vi "Load Normalised ROI setup values file.vi"(11 "Experiment data folder path":path) -> (1 "Normalised ROI file data size":i32[](array[numeric]), 2 "Normalised ROI file data (header removed)":dbl[][](array[numeric]), 3 "Norm ROI columns header":string[](array[string]), 5 "Version index (-1 = latest version)":i32)   [LabVIEW 2017]
uses:
  Typedefs/Enum-Which file or folder.ctl
  <userlib>/My Palettes.lib/Files & paths/Spreadsheet/Read From Spreadsheet File (string)-Mod.vi
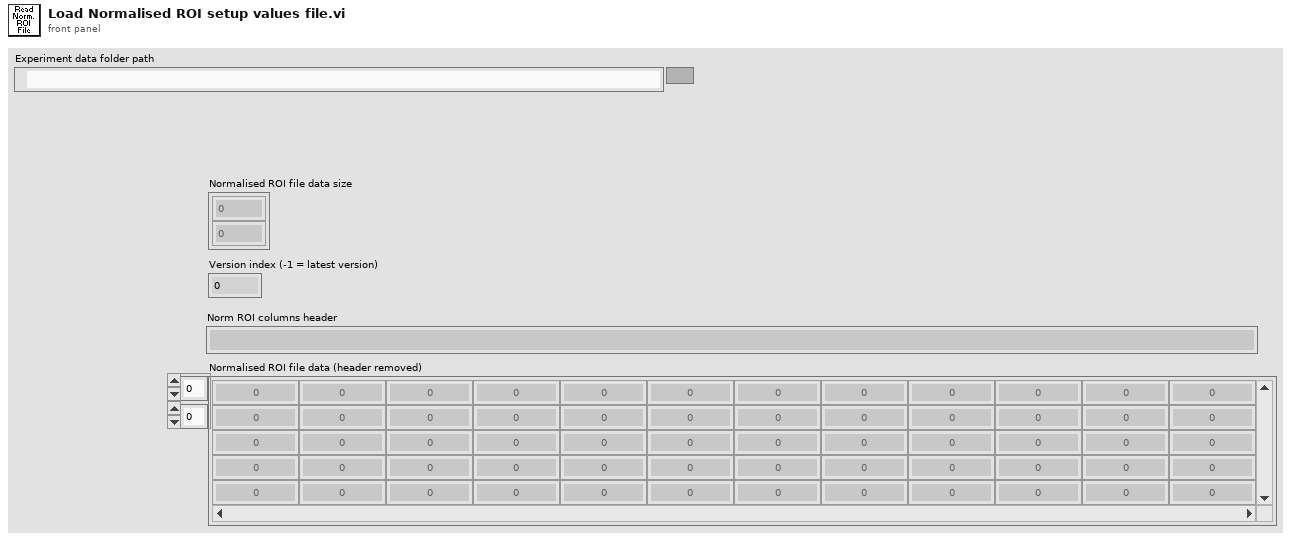
[diagram p1: front panel]
types:
  T1 = typedef "Enum-Which file or folder.ctl" = enum16{"ROI file", "Normalised ROI file", "Zplane Pockels values file", "Functional data folder"}
  T2 = typedef "Fixed strings.ctl" = cluster{"ROI file name":string, "Normalised ROI file name":string, "Zplane Pockels values file name":string, "Functional data folder name":string, "Experiment Header file name":string, "Z-stack images folder name":string, "Groups setup rel. path":string, "Groups text file rel. path":string, "TDMS files folder name (F.img)":string, "TDMS files folder name (V.acq)":string, "TDMS files folder name (Pl.acq)":string, "Cycle rel times sequence file":string, "Dynamically called VIs folder name":string, "Time Series folder base name":string}
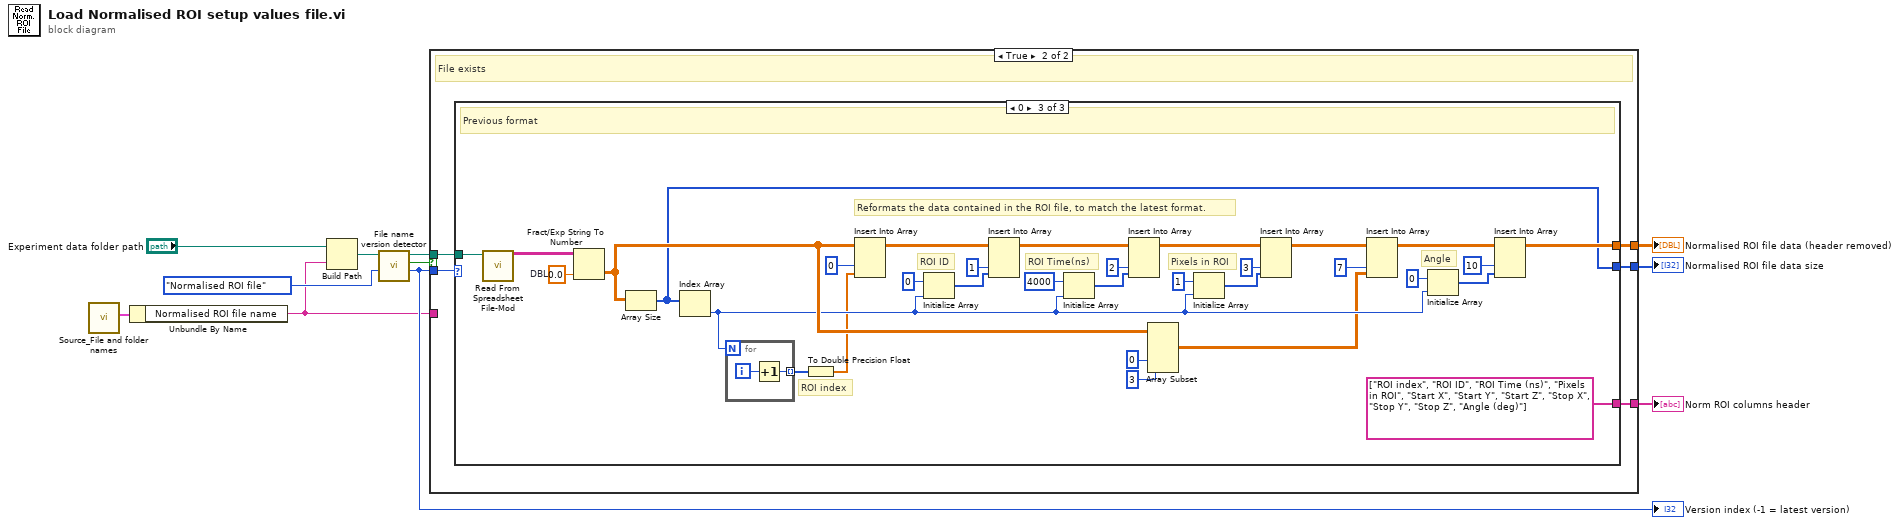
[diagram p0: block diagram]
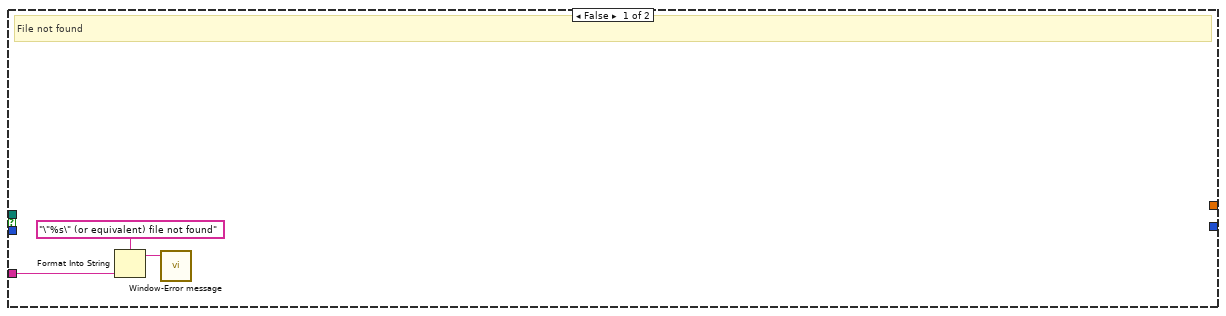
[diagram p2: hidden frame]
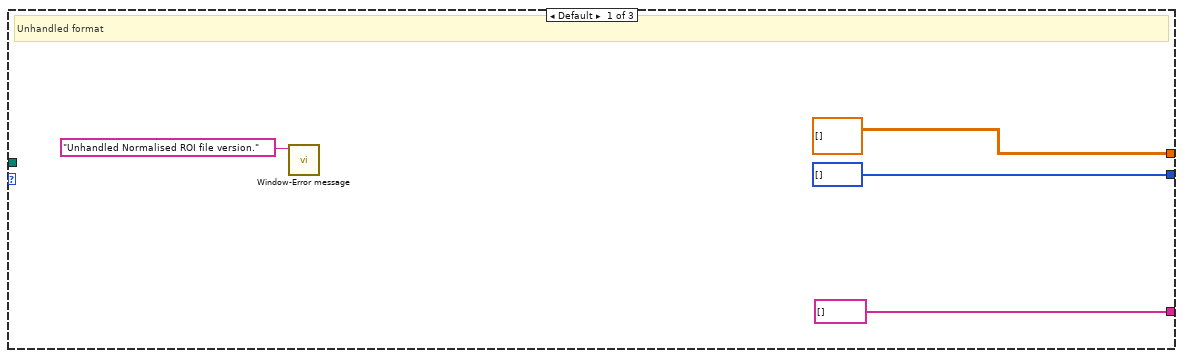
[diagram p3: hidden frame]
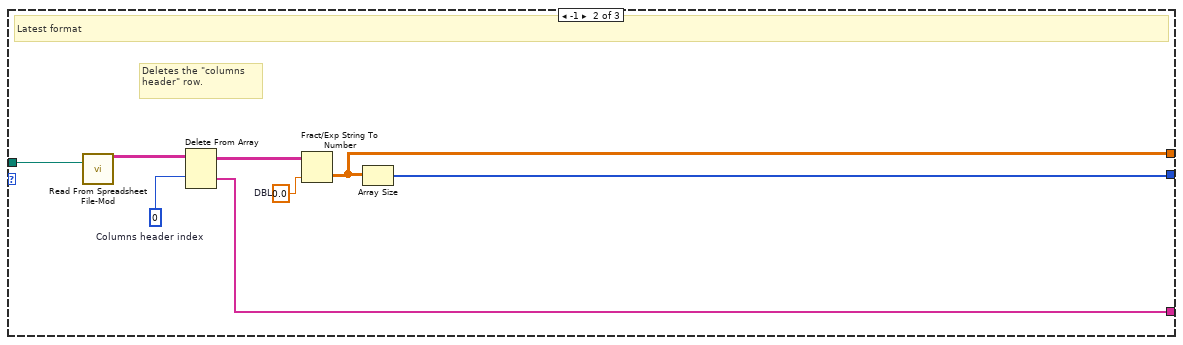
[diagram p4: hidden frame]
diagram:
  n1 = call "Source_File and folder names.vi"() -> ("Fixed strings"=w1:T2)  [unwired: 1 in]
  n2 = Unbundle By Name(w1) -> ("Normalised ROI file name"=w2:string)
  n3 = Build Path(base path="Experiment data folder path", name or relative path=w2) -> (appended path=w11:path)
  n4 = call "File name version detector.vi"("Which file/folder?"=Enum-Which_file_or_folder."Normalised ROI file", "Path in"=w11) -> ("Version index (-1 = latest version)"=w9:i32, "file or folder exists"=w8:bool, "Path out"=w10:path)  [unwired: 7 in]
  "Version index (-1 = latest version)" <- w9
  n5 = case shown="True" w8 {
    tunnel: [_ w19] -> w6
    tunnel: w10 -> [_ w18]
    tunnel: w9 -> [_ w17]
    tunnel: [_ w16] -> w5
    tunnel: w2 -> [w13 _]
    tunnel: [_ w15] -> w4
    frame False {
      # "File not found"
      n6 = Format Into String(format string="\"%s\" (or equivalent) file not found" ("message"), w13) -> (resulting string=w12:string)  [unwired: 2 in, 1 out]
      n7 = call "Window-Error message.vi"("Message"=w12) -> ()  [unwired: 10 in, 1 out]
    }
    frame True {
      # "File exists"
      n8 = case shown="0" w17 {
        tunnel: [dbl[][] [] w28 w35] -> w19
        tunnel: w18 -> [_ w26 w36]
        tunnel: [string[] [] ("all rows") w27 string[] ["ROI index", "ROI ID", "ROI Time (ns)", "Pixels in ROI", "Start X", "Start Y", "Start Z", "Stop X", "Stop Y", "Stop Z", "Angle (deg)"] ("all rows")] -> w16
        tunnel: [i32[] [] w25 w33] -> w15
        frame Default {
          # "Unhandled format"
          n9 = call "Window-Error message.vi"("Message"="Unhandled Normalised ROI file version." ("message")) -> ()  [unwired: 10 in, 1 out]
        }
        frame -1 {
          w29 = 0  # Columns header index
          w30 = 0.0  # DBL
          # "Deletes the \"columns header\" row."
          # "Latest format"
          n10 = call-poly <userlib>:"Read From Spreadsheet File-Mod.vi"("file path (dialog if empty)"=w26) -> ("all rows"=w24:string[][])  [unwired: 9 in, 5 out]
          n11 = Delete From Array(array=w24, index (row)=w29) -> (deleted portion=w27:string[], array with subset deleted=w31:string[][])  [unwired: 2 in]
          n12 = Fract/Exp String To Number(string=w31, default (0 dbl)=w30) -> (number=w28:dbl[][])  [unwired: 2 in, 1 out]
          n13 = Array Size(array=w28) -> (size(s)=w25:i32[])
        }
        frame 0 {
          w37 = 0.0  # DBL
          # "Reformats the data contained in the ROI file, to match the latest format."
          # "Pixels in ROI"
          # "Angle"
          # "ROI Time(ns)"
          # "ROI ID"
          # "ROI index"
          # "Previous format"
          n14 = call-poly <userlib>:"Read From Spreadsheet File-Mod.vi"("file path (dialog if empty)"=w36) -> ("all rows"=w32:string[][])  [unwired: 9 in, 5 out]
          n15 = Fract/Exp String To Number(string=w32, default (0 dbl)=w37) -> (number=w62:dbl[][])  [unwired: 2 in, 1 out]
          n16 = Array Size(array=w62) -> (size(s)=w33:i32[])
          n17 = Index Array(array=w33) -> (element=w61:i32)  [unwired: 1 in]
          n18 = for {
            N: w61 -> [_]
            tunnel: [w64] -> w38 mode=indexing
            i -> [w65]
            n19 = Increment(x=w65) -> (x+1=w64:i32)
          }
          n20 = To Double Precision Float(number=w38) -> (double precision float=w39:dbl[])
          n21 = Insert Into Array "Insert Into Array"(array=w62, index (col)=0 ("disabled index (col)"), new element=w39) -> (w41:dbl[][])  [unwired: 1 in]
          n22 = Initialize Array(i64 0 ("element"), w61) -> (w42:i64[])
          n23 = Insert Into Array "Insert Into Array"(array=w41, index (col)=1 ("disabled index (col)"), new element=w42) -> (w47:dbl[][])  [unwired: 1 in]
          n24 = Initialize Array(i64 4000 ("element"), w61) -> (w45:i64[])
          n25 = Insert Into Array "Insert Into Array"(array=w47, index (col)=2 ("disabled index (col)"), new element=w45) -> (w59:dbl[][])  [unwired: 1 in]
          n26 = Array Subset(array=w62, index (col)=0 ("index (row)"), length (col)=3 ("length")) -> (w51:dbl[][])  [unwired: 2 in]
          n27 = Initialize Array(i64 1 ("element"), w61) -> (w57:i64[])
          n28 = Insert Into Array "Insert Into Array"(array=w59, index (col)=3 ("disabled index (col)"), new element=w57) -> (w60:dbl[][])  [unwired: 1 in]
          n29 = Insert Into Array "Insert Into Array"(array=w60, index (col)=7 ("disabled index (col)"), new element=w51) -> (w53:dbl[][])  [unwired: 1 in]
          n30 = Initialize Array(i64 0 ("element"), w61) -> (w54:i64[])
          n31 = Insert Into Array "Insert Into Array"(array=w53, index (col)=10 ("disabled index (col)"), new element=w54) -> (w35:dbl[][])  [unwired: 1 in]
        }
      }
    }
  }
  "Normalised ROI file data (header removed)" <- w6
  "Normalised ROI file data size" <- w4
  "Norm ROI columns header" <- w5
